vi "Log My Data CSV.vi"(4 "Data element":T1, 8 "error in":errorcluster, 11 "file refnum":refnum<file>) -> (0 "error out":errorcluster, 3 "file refnum out":refnum<file>)   [LabVIEW 2014]
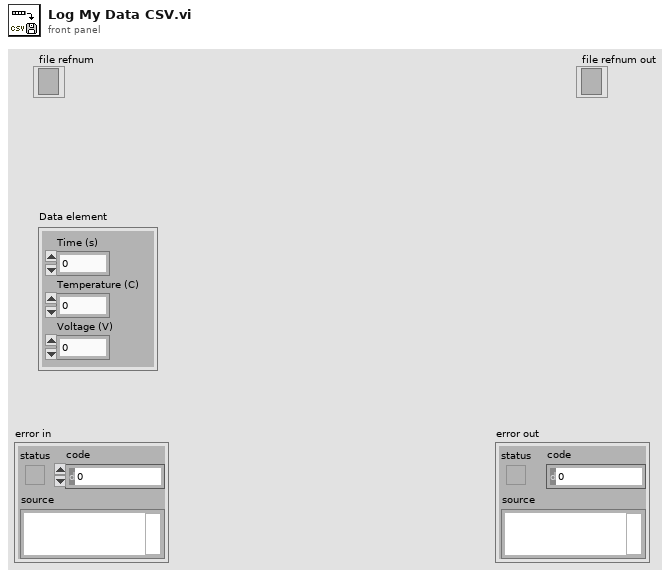
[diagram p1: front panel]
types:
  T1 = cluster{"Time (s)":dbl, "Temperature (C)":dbl, "Voltage (V)":dbl}
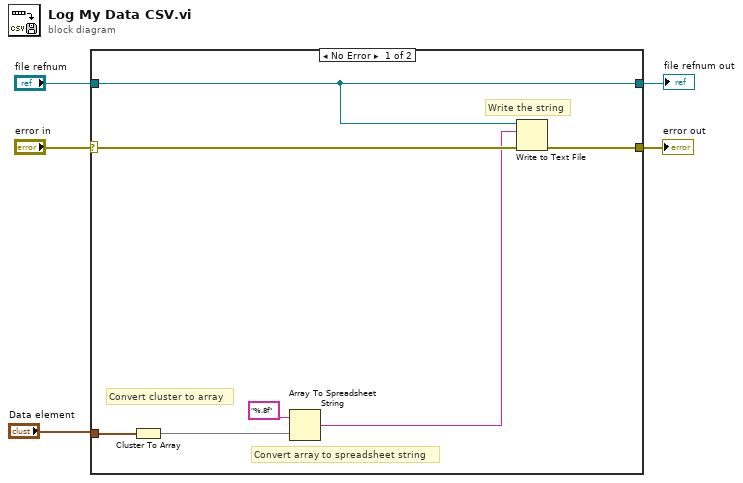
[diagram p0: block diagram]
diagram:
  n1 = case shown="No Error" "error in" {
    selector: "error in" -> [w8 w14]
    tunnel: "Data element" -> [w11 _]
    tunnel: [w9 w14] -> w5
    tunnel: "file refnum" -> [w7 w13]
    tunnel: [w7 w13] -> w1
    frame No Error {
      # "Write the string"
      # "Convert array to spreadsheet string"
      # "Convert cluster to array"
      n2 = Cluster To Array(cluster=w11) -> (array=w10:dbl[])
      n3 = Array To Spreadsheet String(array=w10, 3:"%.8f" ("format string")) -> (spreadsheet string=w6:string)  [unwired: 1 in]
      n4 = Write to Text File(file (use dialog)=w7, text=w6, error in=w8) -> (error out=w9:errorcluster)  [unwired: 1 in, 2 out]
    }
    frame Error {
      # "Wire previous error through"
    }
  }
  "error out" <- w5
  "file refnum out" <- w1
